vi "SENS_CORR_COLL_SESS_SAVE.vi"(0 "VISA IN":refnum<visa-resource-name>, 5 "error in":errorcluster, 7 "Channel":i32, 9 "Session":i32) -> (14 "VISA Out":refnum<visa-resource-name>, 19 "error out":errorcluster)   [LabVIEW 2018, in "PNA-X.lvlib"]
doc: "SENS:CORR:COLL:SESS6:SAVE?"
uses:
  PNA-X.lvlib
panel:
  out "read buffer":string
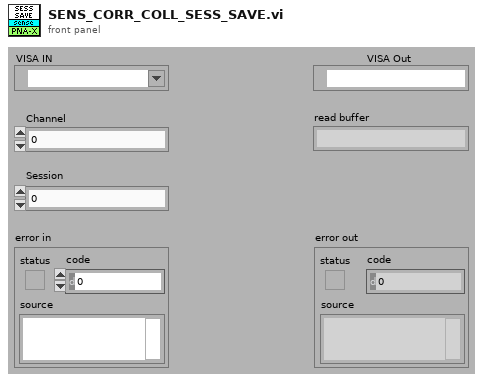
[diagram p1: front panel]
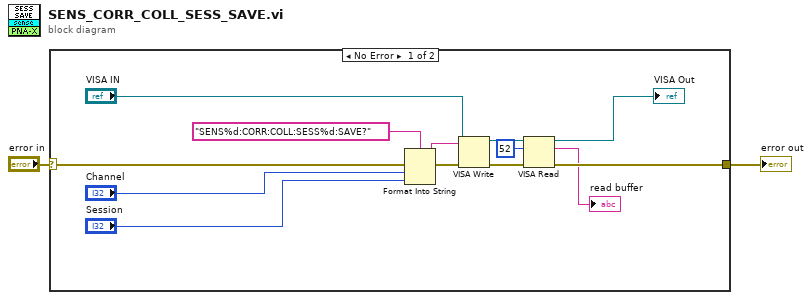
[diagram p0: block diagram]
diagram:
  n1 = case shown="No Error" "error in" {
    selector: "error in" -> [w15 w16]
    tunnel: [w4 w16] -> w1
    frame No Error {
      n2 = Format Into String(format string="SENS%d:CORR:COLL:SESS%d:SAVE?" ("Cmdline"), error in=w15, "Channel", "Session") -> (resulting string=w13:string, error out=w14:errorcluster)  [unwired: 1 in]
      n3 = VISA Write(VISA resource name="VISA IN", write buffer=w13, error in (no error)=w14) -> (VISA resource name out=w8:refnum<visa-resource-name>, error out=w7:errorcluster)  [unwired: 1 out]
      n4 = VISA Read(VISA resource name=w8, byte count=u32 52, error in (no error)=w7) -> (VISA resource name out=→"VISA Out":refnum<visa-resource-name>, read buffer=→"read buffer":string, error out=w4:errorcluster)  [unwired: 1 out]
    }
    frame Error {
    }
  }
  "error out" <- w1
